vi "表格初始化.vi"(10 "设备明细簇":refnum<vi>, 11 "Table输入":refnum<vi>) -> ()   [LabVIEW 2017]
uses:
  <vilib>/Utility/miscctls.llb/LVRowAndColumnTypeDef.ctl
  <vilib>/Utility/miscctls.llb/LVRowAndColumnUnsignedTypeDef.ctl
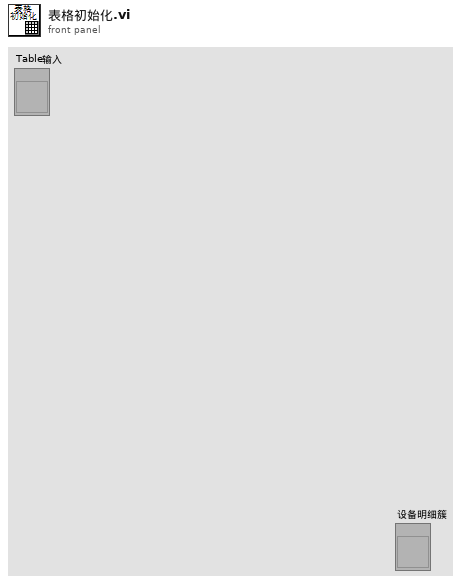
[diagram p1: front panel]
types:
  T1 = typedef "单台设备明细.ctl" = cluster{"设备名称":string, "IP地址":string, "允许开机":bool, "允许连接":bool, "允许归零":bool, "允许自动":bool, "允许退出":bool, "允许关机":bool, "connection ID":refnum<k5>}
  T2 = typedef "LVRowAndColumnUnsignedTypeDef.ctl" = cluster{"Row":u32, "Column":u32}
  T3 = typedef "LVRowAndColumnTypeDef.ctl" = cluster{"Row":i32, "Column":i32}
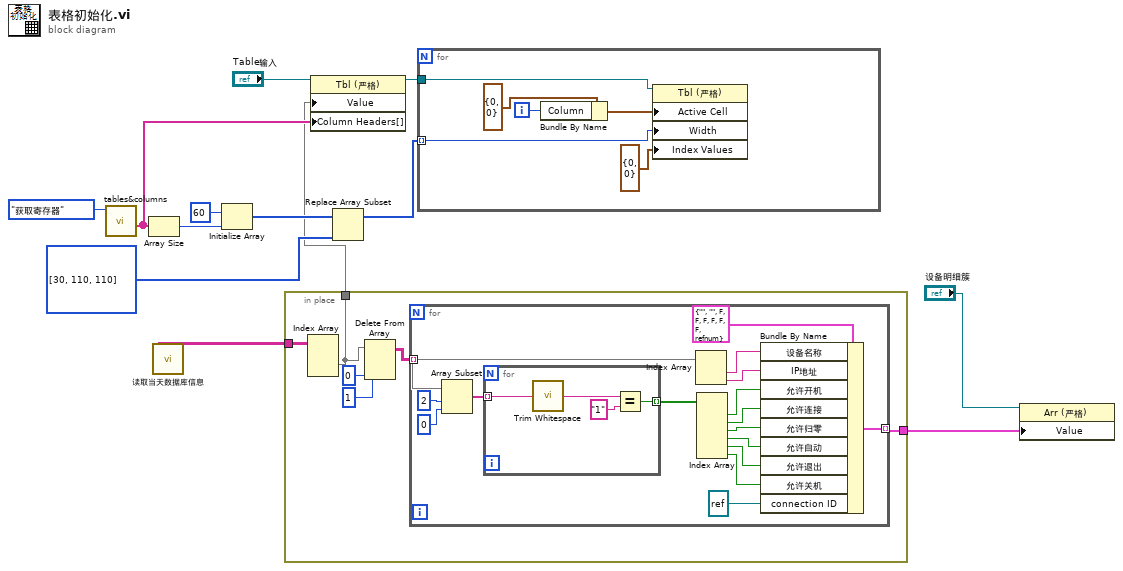
[diagram p0: block diagram]
diagram:
  n1 = call "tables&columns.vi"("选项"=enum16{"初始化", "获取寄存器"}."获取寄存器") -> ("columns"=w10:string[])  [unwired: 9 in, 1 out]
  n2 = Array Size(array=w10) -> (size(s)=w9:i32)
  n3 = call "读取当天数据库信息.vi"() -> ("Results"=w4:string[][][])  [unwired: 11 in]
  n4 = Initialize Array(u32 60 ("元素"), w9) -> (w7:u32[])
  n5 = in-place {
    in-place-border: w4 -> [w19]
    in-place-border: [w17] -> w3
    in-place-border: [w18] -> w2
    n6 = Index Array(array=w19) -> (element=w17:string[][])  [unwired: 3 in]
    n7 = Delete From Array(array=w17, length=1 ("长度"), index (col)=0 ("禁用的索引 (列)")) -> (array with subset deleted=w16:string[][])  [unwired: 1 in, 1 out]
    n8 = for {
      tunnel: w16 -> [w31] mode=indexing
      tunnel: [w28] -> w18 mode=indexing
      n9 = Array Subset(array=w31, index=2 ("索引"), length=0 ("长度")) -> (w27:string[])
      n10 = for {
        tunnel: w27 -> [w39] mode=indexing
        tunnel: [w36] -> w26 mode=indexing
        n11 = call <vilib>:"Trim Whitespace.vi"("string"=w39) -> ("trimmed string"=w38:string)  [unwired: 1 in]
        n12 = Equal?(x=w38, y="1") -> (x = y?=w36:bool)
      }
      n13 = Index Array(array=w31) -> (element #1=w34:string, element #2=w33:string)  [unwired: 2 in]
      n14 = Index Array(array=w26) -> (element #1=w25:bool, element #2=w24:bool, element #3=w23:bool, element #4=w22:bool, element #5=w21:bool, element #6=w20:bool)  [unwired: 6 in]
      n15 = Bundle By Name(cluster=T1 {"设备名称"="", "IP地址"="", "允许开机"=FALSE, "允许连接"=FALSE, "允许归零"=FALSE, "允许自动"=FALSE, "允许退出"=FALSE, "允许关机"=FALSE, "connection ID"=refnum} ("单台设备明细"), "设备名称"=w34, "IP地址"=w33, "允许开机"=w25, "允许连接"=w24, "允许归零"=w23, "允许自动"=w22, "允许退出"=w21, "允许关机"=w20, "connection ID"=refnum<k5> refnum ("connection ID in")) -> (w28:T1)
    }
  }
  n16 = property class="Tbl (严格)"(reference="Table输入", "Value"=w3, "Column Headers[]"=w10) -> (reference out=w11:refnum<vi>)  [unwired: 1 in, 1 out]
  n17 = Replace Array Subset(array=w7, new element=u32[] [30, 110, 110]) -> (w5:u32[])  [unwired: 1 in]
  n18 = for {
    tunnel: w5 -> [w42] mode=indexing
    tunnel: w11 -> [w40]
    i -> [w43]
    n19 = Bundle By Name(cluster=T3 {"Row"=0, "Column"=0} ("活动单元格:活动单元格"), "Column"=w43) -> (w44:T3)
    n20 = property class="Tbl (严格)"(reference=w40, "Active Cell"=w44, "Width"=w42, "Index Values"=T2 {"Row"=0, "Column"=0} ("索引值")) -> ()  [unwired: 1 in, 2 out]
  }
  n21 = property class="Arr (严格)"(reference="设备明细簇", "Value"=w2) -> ()  [unwired: 1 in, 2 out]
